vi "load cvt3 taglist.vi"(10 "cfg file path":path, 11 "vi path":path) -> (2 "ok?":bool, 3 "tags":refnum<class "tag descriptor.lvclass">[](array[class]))   [LabVIEW 2013, in "PL Framework Configuration Tool.lvlib" / "EngineTags.lvclass"]
uses:
  EngineTags.lvclass
  <vilib>/NI/Tag Bus/tag/tag descriptor.lvclass
  <vilib>/NI/Tag Bus/tag/Data Type.ctl
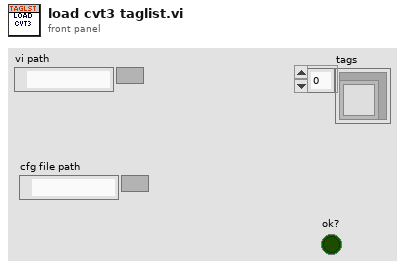
[diagram p1: front panel]
types:
  T1 = cluster{"Tags":cluster{"Data Type":enum16{"Double", "Single", "I64", "I32", "I16", "I8", "U64", "U32", "U16", "U8", "String", "Boolean", "Array of U8", "Array of U16", "Array of U32", "Array of U64", "Array of I64", "Array of I32", "Array of I16", "Array of I8", "Array of Double", "Array of Single", "Array of Boolean", "Array of String"}, "Name":string, "Value":string, "Description":string}[], "Group Listings":cluster{"Group":string, "Tag Names":string[]}[]}
  T2 = cluster{"Data Type":enum16{"Double", "Single", "I64", "I32", "I16", "I8", "U64", "U32", "U16", "U8", "String", "Boolean", "Array of U8", "Array of U16", "Array of U32", "Array of U64", "Array of I64", "Array of I32", "Array of I16", "Array of I8", "Array of Double", "Array of Single", "Array of Boolean", "Array of String"}, "Name":string, "Value":string, "Description":string}[]
  T3 = typedef "tag bus.lvlib/tag descriptor.lvclass/Data Type.ctl" = enum16{"Double", "Single", "I64", "I32", "I16", "I8", "U64", "U32", "U16", "U8", "Boolean", "String", "Array of Double", "Array of Single", "Array of I64", "Array of I32", "Array of I16", "Array of I8", "Array of U64", "Array of U32", "Array of U16", "Array of U8", "Array of Boolean", "Array of String"}
  T4 = enum16{"Double", "Single", "I64", "I32", "I16", "I8", "U64", "U32", "U16", "U8", "String", "Boolean", "Array of U8", "Array of U16", "Array of U32", "Array of U64", "Array of I64", "Array of I32", "Array of I16", "Array of I8", "Array of Double", "Array of Single", "Array of Boolean", "Array of String"}
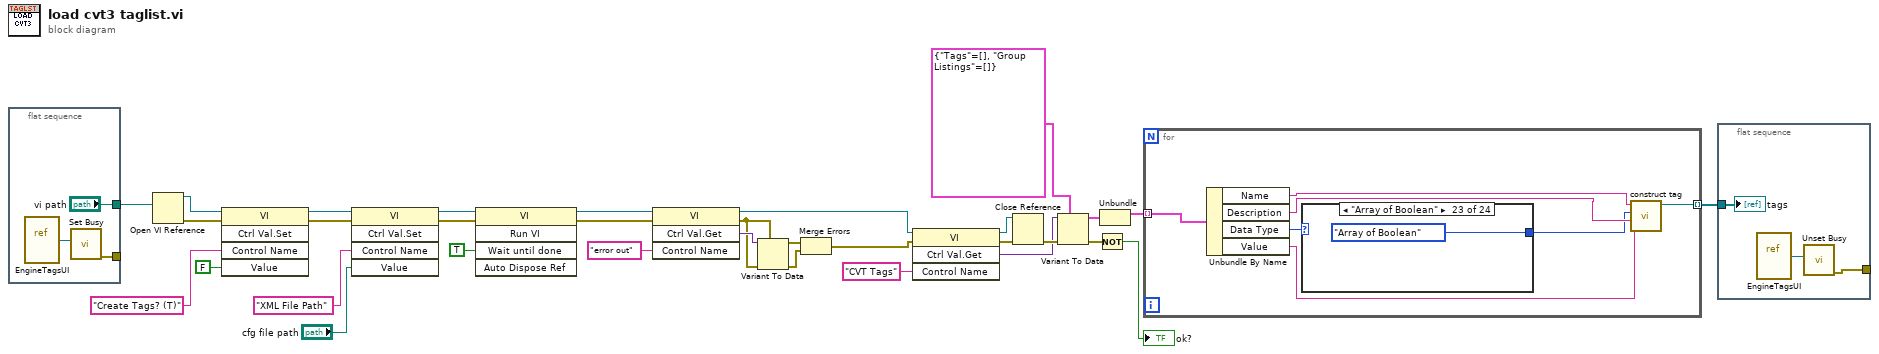
[diagram p0: block diagram]
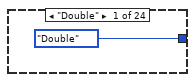
[diagram p2: hidden frame]
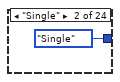
[diagram p3: hidden frame]
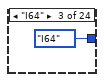
[diagram p4: hidden frame]
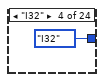
[diagram p5: hidden frame]
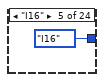
[diagram p6: hidden frame]
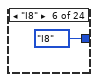
[diagram p7: hidden frame]
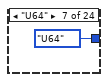
[diagram p8: hidden frame]
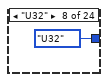
[diagram p9: hidden frame]
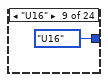
[diagram p10: hidden frame]
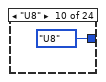
[diagram p11: hidden frame]
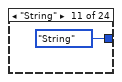
[diagram p12: hidden frame]
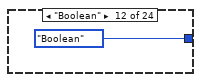
[diagram p13: hidden frame]
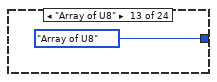
[diagram p14: hidden frame]
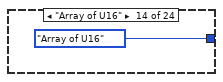
[diagram p15: hidden frame]
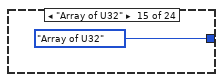
[diagram p16: hidden frame]
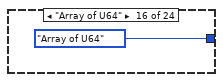
[diagram p17: hidden frame]
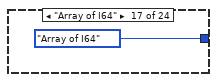
[diagram p18: hidden frame]
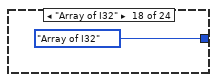
[diagram p19: hidden frame]
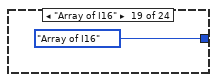
[diagram p20: hidden frame]
diagram:
  n1 = flat-sequence {
    tunnel: [w34] -> _
    tunnel: ["vi path"] -> w2
    frame #0 {
      n2 = vi-ref "EngineTagsUI.vi"() -> (w35:refnum<vi>)
      n3 = call <vilib>:"Set Busy.vi"("VI reference (current VI)"=w35) -> ("error out"=w34:errorcluster)  [unwired: 9 in, 1 out]
    }
  }
  n4 = Open VI Reference(vi path=w2) -> (vi reference=w31:refnum<vi>, error out=w32:errorcluster)  [unwired: 5 in]
  n5 = invoke class="VI" method="Ctrl Val.Set"(reference=w31, error in=w32, "Control Name"="Create Tags? (T)", "Value"=FALSE) -> (reference out=w29:refnum<vi>, error out=w30:errorcluster)  [unwired: 1 in, 3 out]
  n6 = invoke class="VI" method="Ctrl Val.Set"(reference=w29, error in=w30, "Control Name"="XML File Path", "Value"="cfg file path") -> (reference out=w5:refnum<vi>, error out=w27:errorcluster)  [unwired: 1 in, 3 out]
  n7 = invoke class="VI" method="Run VI"(reference=w5, error in=w27, "Wait until done"=TRUE ("Wait Until Done")) -> (reference out=w4:refnum<vi>, error out=w6:errorcluster)  [unwired: 2 in, 3 out]
  n8 = invoke class="VI" method="Ctrl Val.Get"(reference=w4, error in=w6, "Control Name"="error out") -> (reference out=w28:refnum<vi>, error out=w20:errorcluster, "Get Control Value Variant"=w21:variant)  [unwired: 1 in, 1 out]
  n9 = Variant To Data(error in=w20, type=w20, Variant=w21) -> (data=w18:errorcluster, error out=w22:errorcluster)
  n10 = Merge Errors(w18, w22) -> (w19:errorcluster)
  n11 = invoke class="VI" method="Ctrl Val.Get"(reference=w28, error in=w19, "Control Name"="CVT Tags") -> (reference out=w14:refnum<vi>, error out=w16:errorcluster, "Get Control Value Variant"=w12:variant)  [unwired: 1 in, 1 out]
  n12 = Close Reference(reference=w14, error in (no error)=w16) -> (error out=w15:errorcluster)
  n13 = Variant To Data(error in=w15, type=T1 {"Tags"=[], "Group Listings"=[]} ("CVT Tags"), Variant=w12) -> (data=w10:T1, error out=w13:errorcluster)
  n14 = Not(x=w13) -> (.not. x?=→"ok?":bool)
  n15 = Unbundle(w10) -> ("Tags"=w7:T2)  [unwired: 1 out]
  n16 = for {
    tunnel: w7 -> [w42] mode=indexing
    tunnel: [w36] -> w1 mode=indexing
    n17 = Unbundle By Name(w42) -> ("Name"=w40:string, "Description"=w39:string, "Data Type"=w41:T4, "Value"=w37:string)
    n18 = case shown="\"Array of Boolean\"" w41 {
      tunnel: [Data_Type."Double" ("Expected Type") Data_Type."Single" ("Expected Type") Data_Type."I64" ("Expected Type") Data_Type."I32" ("Expected Type") Data_Type."I16" ("Expected Type") Data_Type."I8" ("Expected Type") Data_Type."U64" ("Expected Type") Data_Type."U32" ("Expected Type") Data_Type."U16" ("Expected Type") Data_Type."U8" ("Expected Type") Data_Type."String" ("Expected Type") Data_Type."Boolean" ("Expected Type") Data_Type."Array of U8" ("Expected Type") Data_Type."Array of U16" ("Expected Type") Data_Type."Array of U32" ("Expected Type") Data_Type."Array of U64" ("Expected Type") Data_Type."Array of I64" ("Expected Type") Data_Type."Array of I32" ("Expected Type") Data_Type."Array of I16" ("Expected Type") Data_Type."Array of I8" ("Expected Type") Data_Type."Array of Double" ("Expected Type") Data_Type."Array of Single" ("Expected Type") Data_Type."Array of Boolean" ("Expected Type") Data_Type."Array of String" ("Expected Type")] -> w38
      frame "Double" {
      }
      frame "Single" {
      }
      frame "I64" {
      }
      frame "I32" {
      }
      frame "I16" {
      }
      frame "I8" {
      }
      frame "U64" {
      }
      frame "U32" {
      }
      frame "U16" {
      }
      frame "U8" {
      }
      frame "String" {
      }
      frame "Boolean" {
      }
      frame "Array of U8" {
      }
      frame "Array of U16" {
      }
      frame "Array of U32" {
      }
      frame "Array of U64" {
      }
      frame "Array of I64" {
      }
      frame "Array of I32" {
      }
      frame "Array of I16" {
      }
      frame "Array of I8" {
      }
      frame "Array of Double" {
      }
      frame "Array of Single" {
      }
      frame "Array of Boolean" {
      }
      frame "Array of String" {
      }
    }
    n19 = call <vilib>:"construct tag.vi"("raw default"=w37, "metadata"=w39, "data type"=w38, "name"=w40) -> ("system tag out"=w36:refnum<class "tag descriptor.lvclass">)  [unwired: 6 in, 1 out]
  }
  n20 = flat-sequence {
    tunnel: [w68] -> _
    tunnel: w1 -> [w67]
    frame #0 {
      n21 = vi-ref "EngineTagsUI.vi"() -> (w69:refnum<vi>)
      n22 = call <vilib>:"Unset Busy.vi"("VI reference (current VI)"=w69) -> ("error out"=w68:errorcluster)  [unwired: 10 in]
      "tags" <- w67
    }
  }
